vi "ConfigureChannels.vi"(8 "error in (no error)":errorcluster, 11 "NIScope in":refnum<class "NIScope.lvclass">) -> (0 "error out":errorcluster, 3 "NIScope out":refnum<class "NIScope.lvclass">)   [LabVIEW 2014, in "ScopePlugins.lvlib" / "NIScope.lvclass"]
uses:
  NIScope.lvclass
  TypeDefs/Channels.ctl
  TypeDefs/Channel.ctl
  ScopePluginBaseClass/ScopePluginsBase.lvclass/ScopePluginsBase.ctl
  ScopePluginBaseClass/Accessors/Read Channels.vi
  ScopePluginBaseClass/Accessors/Write Channels.vi
  ScopePlugins.lvlib
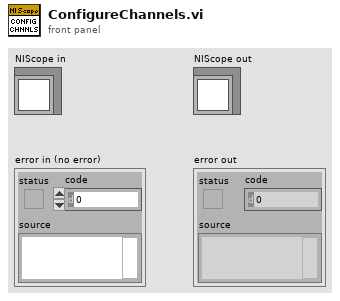
[diagram p1: front panel]
types:
  T1 = cluster{"instrument handle":refnum<k15>, string}[]
  T2 = typedef "ScopePlugins.lvlib/Channels.ctl" = cluster{"Count":i32, "ChannelArray":T3[]}
  T3 = typedef "ScopePlugins.lvlib/Channel.ctl" = cluster{"Enabled":bool, "Name":string, "InputImpedance":dbl, "InputFreqMax":dbl, "ProbeAttn":dbl, "Coupling":enum16{"AC", "DC", "GND"}, "Offset":dbl, "Range":dbl, "Handle":string, "Connected":bool}
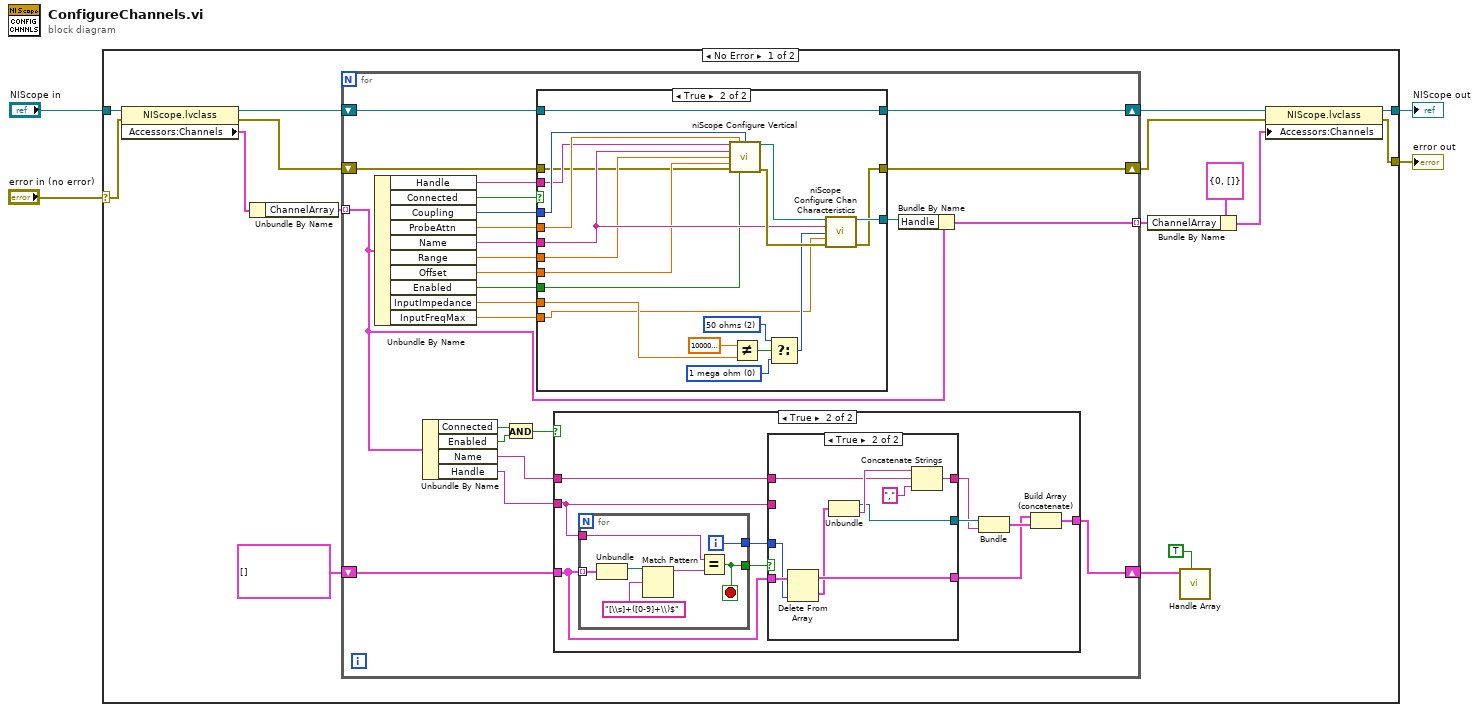
[diagram p0: block diagram]
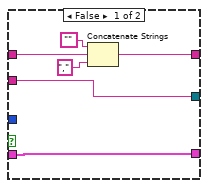
[diagram p3: hidden frame]
diagram:
  n1 = case shown="No Error" "error in (no error)" {
    selector: "error in (no error)" -> [w19 w101]
    tunnel: "NIScope in" -> [w20 w102]
    tunnel: [w13 w102] -> w2
    tunnel: [w8 w101] -> w1
    frame No Error {
      n2 = property class="NIScope.lvclass"(reference=w20, error in=w19) -> (reference out=w18:refnum<class "NIScope.lvclass">, error out=w17:errorcluster, "Accessors:Channels"=w15:T2)
      n3 = Unbundle By Name(w15) -> ("ChannelArray"=w14:T3[])
      n4 = for {
        shift-right: [w30] -> w16
        shift-left: w18 -> [w44]
        shift-right: [w42] -> w9
        shift-left: w17 -> [w43]
        tunnel: w14 -> [w23] mode=indexing
        tunnel: [w29] -> w11 mode=indexing
        shift-right: [w21] -> w6
        shift-left: T1 [] -> [w22]
        n5 = Unbundle By Name(w23) -> ("Handle"=w32:string, "Connected"=w41:bool, "Coupling"=w40:enum16{"AC", "DC", "GND"}, "ProbeAttn"=w39:dbl, "Name"=w38:string, "Range"=w37:dbl, "Offset"=w36:dbl, "Enabled"=w35:bool, "InputImpedance"=w34:dbl, "InputFreqMax"=w33:dbl)
        n6 = Unbundle By Name(w23) -> ("Connected"=w25:bool, "Enabled"=w26:bool, "Name"=w28:string, "Handle"=w27:string)
        n7 = And(x=w25, y=w26) -> (x .and. y?=w24:bool)
        n8 = case shown="True" w41 {
          tunnel: w44 -> [w79 w81]
          tunnel: w43 -> [w80 w84]
          tunnel: [w80 w82] -> w42
          tunnel: w40 -> [_ w93]
          tunnel: w39 -> [_ w92]
          tunnel: w38 -> [_ w91]
          tunnel: w37 -> [_ w90]
          tunnel: w36 -> [_ w89]
          tunnel: w35 -> [_ w88]
          tunnel: w34 -> [_ w87]
          tunnel: w33 -> [_ w86]
          tunnel: w32 -> [w78 w85]
          tunnel: [w78 w83] -> w31
          tunnel: [w79 w81] -> w30
          frame False {
          }
          frame True {
            w95 = u32 0 items=["1 mega ohm"=0, "50 ohms"=2] ("input impedance")
            w96 = u32 2 items=["1 mega ohm"=0, "50 ohms"=2] ("input impedance")
            n9 = call <instrlib>:"niScope Configure Vertical.vi"("instrument handle"=w85, "probe attenuation"=w92, "vertical coupling"=w93, "channels"=w91, "vertical range"=w90, "vertical offset"=w89, "error in"=w84, "channel enabled"=w88) -> ("instrument handle out"=w99:refnum<k15>, "error out"=w100:errorcluster)  [unwired: 6 in]
            n10 = Not Equal?(x=1000000.0, y=w87) -> (x != y?=w98:bool)
            n11 = Select(t=w96, s=w98, f=w95) -> (s? t:f=w94:u32)
            n12 = call <instrlib>:"niScope Configure Chan Characteristics.vi"("instrument handle"=w99, "channels"=w91, "input impedance"=w94, "maximum input frequency"=w86, "error in"=w100) -> ("instrument handle out"=w83:refnum<k15>, "error out"=w82:errorcluster)  [unwired: 9 in]
          }
        }
        n13 = case shown="True" w24 {
          tunnel: w28 -> [_ w52]
          tunnel: w22 -> [w45 w49]
          tunnel: w27 -> [_ w53]
          tunnel: [w45 w54] -> w21
          frame False {
          }
          frame True {
            n14 = for {
              tunnel: w49 -> [w74] mode=indexing
              tunnel: w53 -> [w75]
              tunnel: [w72] -> w55
              tunnel: [w71] -> w51
              i -> [w71]
              stop <- w72 stop-if-true
              n15 = Unbundle(w74) -> ("instrument handle"=w73:refnum<k15>)  [unwired: 1 out]
              n16 = Match Pattern(string=w73, regular expression="[\\s]+([0-9]+\\)$") -> (before substring=w76:string)  [unwired: 1 in, 3 out]
              n17 = Equal?(x=w75, y=w76) -> (x = y?=w72:bool)
            }
            n18 = case shown="True" w55 {
              tunnel: w53 -> [w60 _]
              tunnel: w52 -> [w59 w65]
              tunnel: [w61 w62] -> w46
              tunnel: [w60 w63] -> w47
              tunnel: w51 -> [_ w68]
              tunnel: w49 -> [w57 w70]
              tunnel: [w57 w69] -> w48
              frame False {
                n19 = Concatenate Strings("", w59, ",") -> (w61:string)
              }
              frame True {
                n20 = Delete From Array(array=w70, index=w68) -> (deleted portion=w67:cluster{"instrument handle":refnum<k15>, string}, array with subset deleted=w69:T1)  [unwired: 1 in]
                n21 = Unbundle(w67) -> ("instrument handle"=w63:refnum<k15>, w66:string)
                n22 = Concatenate Strings(w66, w65, "," ("string")) -> (w62:string)
              }
            }
            n23 = Bundle("instrument handle"=w47, w46) -> (w50:cluster{"instrument handle":refnum<k15>, string})  [unwired: 1 in]
            n24 = Build Array (concatenate)(w48, w50) -> (w54:T1)
          }
        }
        n25 = Bundle By Name(cluster=w23, "Handle"=w31) -> (w29:T3)
      }
      n26 = Bundle By Name(cluster=T2 {"Count"=0, "ChannelArray"=[]} ("Channels"), "ChannelArray"=w11) -> (w10:T2)
      n27 = call "Handle Array.vi"("Set(f)"=TRUE, "Array Handles"=w6) -> ()  [unwired: 9 in, 1 out]
      n28 = property class="NIScope.lvclass"(reference=w16, error in=w9, "Accessors:Channels"=w10) -> (reference out=w13:refnum<class "NIScope.lvclass">, error out=w8:errorcluster)
    }
    frame Error {
    }
  }
  "error out" <- w1
  "NIScope out" <- w2
